vi "GMLAN CloseConnection.vi"(8 "error in (no error)":errorcluster, 10 "diag ref out":T2, 11 "UUDT Engine":T1) -> (0 "error out":errorcluster)   [LabVIEW 2013, in "GMLAN.lvlib"]
uses:
  GMLAN.lvlib
  <vilib>/Automotive Diagnostic Command Set/Diagnostic Transport.llb/Diag Reference.ctl
  <vilib>/Automotive Diagnostic Command Set/Diagnostic Transport.llb/Transport Protocol Selector.ctl
  <vilib>/Automotive Diagnostic Command Set/Diagnostic Transport.llb/Diag CAN Frame Log.ctl
  _SubVIs/UUDT Engine Refs.ctl
  _SubVIs/UUDT Engine Connection List_Action.ctl
  <vilib>/addons/Automotive Diagnostic Command Set/NI_Automotive Diagnostic Command Set.lvlib
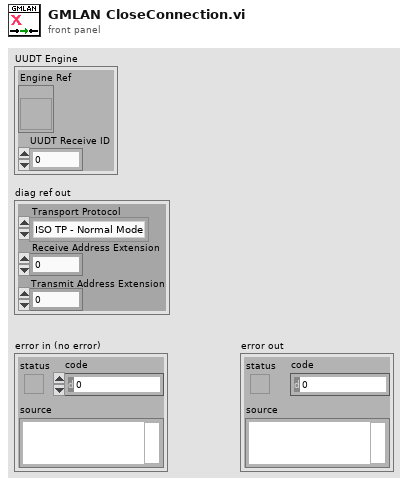
[diagram p1: front panel]
types:
  T1 = typedef "GMLAN.lvlib/UUDT Engine Refs.ctl" = cluster{"Engine Ref":refnum<vi>, "UUDT Receive ID":u32}
  T2 = typedef "NI_Automotive Diagnostic Command Set.lvlib/Diag Reference.ctl" = cluster{"Diag CAN Handle":u32, "Transport Protocol":T3, "Receive Address Extension":u8, "Transmit Address Extension":u8, "Receive CAN Id":u32, "Transmit CAN Id":u32, "Diag CAN Queue":refnum<queue>, "Log Frames ?":bool, "My TP Address":u8, "Other TP Address":u8, "T1":u16, "T2":u16, "T3":u16, "T4":u16, "Tx SN":u8, "Block Size":u8, "Rx SN":u8, "VW TP Initialized?":bool, "Tx block no":u8, "baud rate":u32, "Interface":string, "Channel Diag CAN Handle":u32, "UDP Connection ID":refnum<k16>, "TCP Connection ID":refnum<k5>, "Target IP Addr":u32, "Source Address":u16, "Target Address":u16, "Send Header NACK?":bool, "DLL Handle":u32, "NAD":u8}
  T3 = typedef "NI_Automotive Diagnostic Command Set.lvlib/Transport Protocol Selector.ctl" = enum16{"ISO TP - Normal Mode", "ISO TP - Mixed Mode", "VW TP 2.0", "Diagnostics on IP", "ISO TP LIN"}
  T4 = typedef "GMLAN.lvlib/UUDT Engine Connection List_Action.ctl" = enum8{"Initialize", "Write", "Add", "Read"}
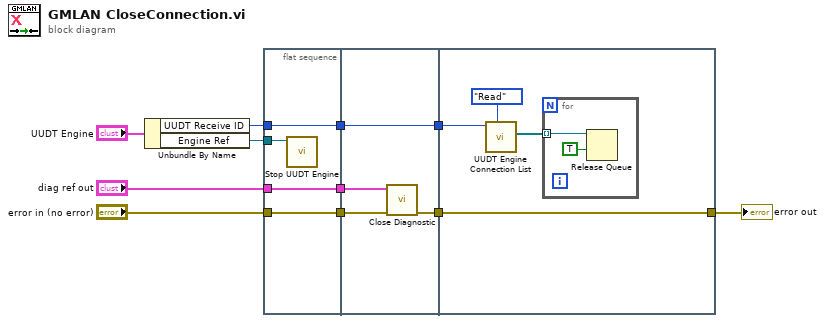
[diagram p0: block diagram]
diagram:
  n1 = Unbundle By Name("UUDT Engine") -> ("UUDT Receive ID"=w3:u32, "Engine Ref"=w5:refnum<vi>)
  n2 = flat-sequence {
    tunnel: [w15] -> w11
    tunnel: "error in (no error)" -> [w15]
    tunnel: [w14] -> w8
    tunnel: "diag ref out" -> [w14]
    tunnel: w5 -> [w13]
    tunnel: w3 -> [w12]
    tunnel: [w12] -> w1
    tunnel: w11 -> [w19]
    tunnel: w8 -> [w17]
    tunnel: [w18] -> w4
    tunnel: [w16] -> w2
    tunnel: w1 -> [w16]
    tunnel: [w23] -> w9
    tunnel: w4 -> [w23]
    tunnel: w2 -> [w22]
    frame #0 {
      n3 = call "Stop UUDT Engine.vi"("vi reference"=w13) -> ()  [unwired: 11 in]
    }
    frame #1 {
      n4 = call <vilib>:"Close Diagnostic.vi"("error in (no error)"=w19, "diag ref in"=w17) -> ("error out"=w18:errorcluster)  [unwired: 9 out]
    }
    frame #2 {
      n5 = call "UUDT Engine Connection List.vi"("Action"=UUDT_Engine_Connection_List_Action."Read", "UUDT"=w22) -> ("Queue List"=w20:refnum<queue>[])  [unwired: 8 in, 1 out]
      n6 = for {
        tunnel: w20 -> [w25] mode=indexing
        n7 = Release Queue(queue=w25, force destroy? (F)=TRUE) -> ()  [unwired: 1 in, 3 out]
      }
    }
  }
  "error out" <- w9
